vi "niFpgaMeanVarStdOutsideSCTL.vi"(0 "input data":fxp<+/-,32,1>, 1 "reset":bool) -> (4 "mean":fxp<+/-,32,1> format="%.32g", 6 "standard deviation":fxp<+,32,1> format="%.32g", 8 "variance":fxp<+,63,1> format="%.63g", 10 "output valid":bool)   [LabVIEW 2017]
doc: "Calculates the <B>DC (Mean)</B> and/or <B>RMS</B> values of an input signal. You also can use this VI to calculate the intermediate <B>Sum</B>, <B>Mean Square</B>, and <B>Square Sum</B> values in order to save FPGA resources."
uses:
  <vilib>/rvi/FXPMathLib/basic elements/FxpIntAccumulator/XNode/nifxpmath_IntAccumulator.xnode
  <vilib>/rvi/FXPMathLib/basic elements/FxpIntAccumulator/simVIs/DllFxpIntAccumulator_sub.vi
  <vilib>/rvi/FXPMathLib/basic elements/FxpIntAccumulator/subVIs/nifxpmath_IntAccumulator_SimConfig.ctl
  <vilib>/rvi/FXPMathLib/FxpMul/XNode/nifxpmath_Multiplier.xnode
  <vilib>/fxp/LVFixedPointOverflowPolicyTypeDef.ctl
  <vilib>/rvi/FXPMathLib/FxpSqrt/XNode/nifxpmath_Sqrt.xnode
  <vilib>/Platform/TimedLoop/XDataNode/XDataNode.xnode
  <vilib>/Platform/TimedLoop/XDataNode/nitl_modes.ctl
  <vilib>/Platform/TimedLoop/XDataNode/XDNodeRunTimeDep.lvlib
  <vilib>/Platform/TimedLoop/XDataNode/wakeup.ctl
  <vilib>/Platform/TimedLoop/XDataNode/timing_clust.ctl
  <vilib>/rvi/FXPMathLib/FxpSqrt/simVIs/DllSqrtTemp_sub.vi
  <vilib>/rvi/FXPMathLib/FxpSqrt/subVIs/nifxpmath_Sqrt_SimConfig.ctl
  <vilib>/rvi/FXPMathLib/sim/FxpSim.dll
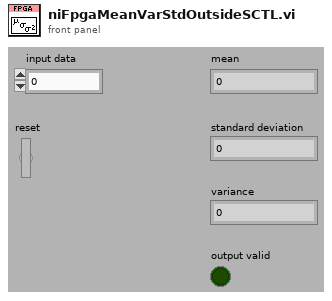
[diagram p1: front panel]
types:
  T1 = typedef "XDNodeRunTimeDep.lvlib/timing_clust.ctl" = cluster{"Expected End [f-1]":u64, "Actual End [f-1]":u64, "Finished Late? [f-1]":bool, "Expected End [i-1]":u64, "Actual End [i-1]":u64, "Finished Late? [i-1]":bool, "Expected Start [i]":u64, "Actual Start [i]":u64, "Expected Start [f]":u64, "Actual Start [f]":u64, "Source Name":string, "Structure Name":string, "Period":i64, "Deadline":i64, "Offset":i64, "Start":i64, "Priority":i32, "Timeout":i32, "Mode":T2, "Wakeup Reason":T3, "Error":errorcluster, "Source Type":string, "Secondary Source Type":string, "Global End Time":u64, "Global Start Time":u64, "Frame Duration":u64, "Iteration Duration":u64, "Assigned CPU":i32, "I/O Scan Engine Mode":u32}
  T2 = typedef "XDNodeRunTimeDep.lvlib/nitl_modes.ctl" = enum32{"No Change", "Process missed periods, maintain original phase", "Discard missed periods, maintain original phase", "Process missed periods, ignore original phase", "Discard missed periods, ignore original phase"}
  T3 = typedef "XDNodeRunTimeDep.lvlib/wakeup.ctl" = enum32{"Normal", "Aborted", "Asynchronous wakeup", "Timing source error", "Timed loop error", "Timeout"}
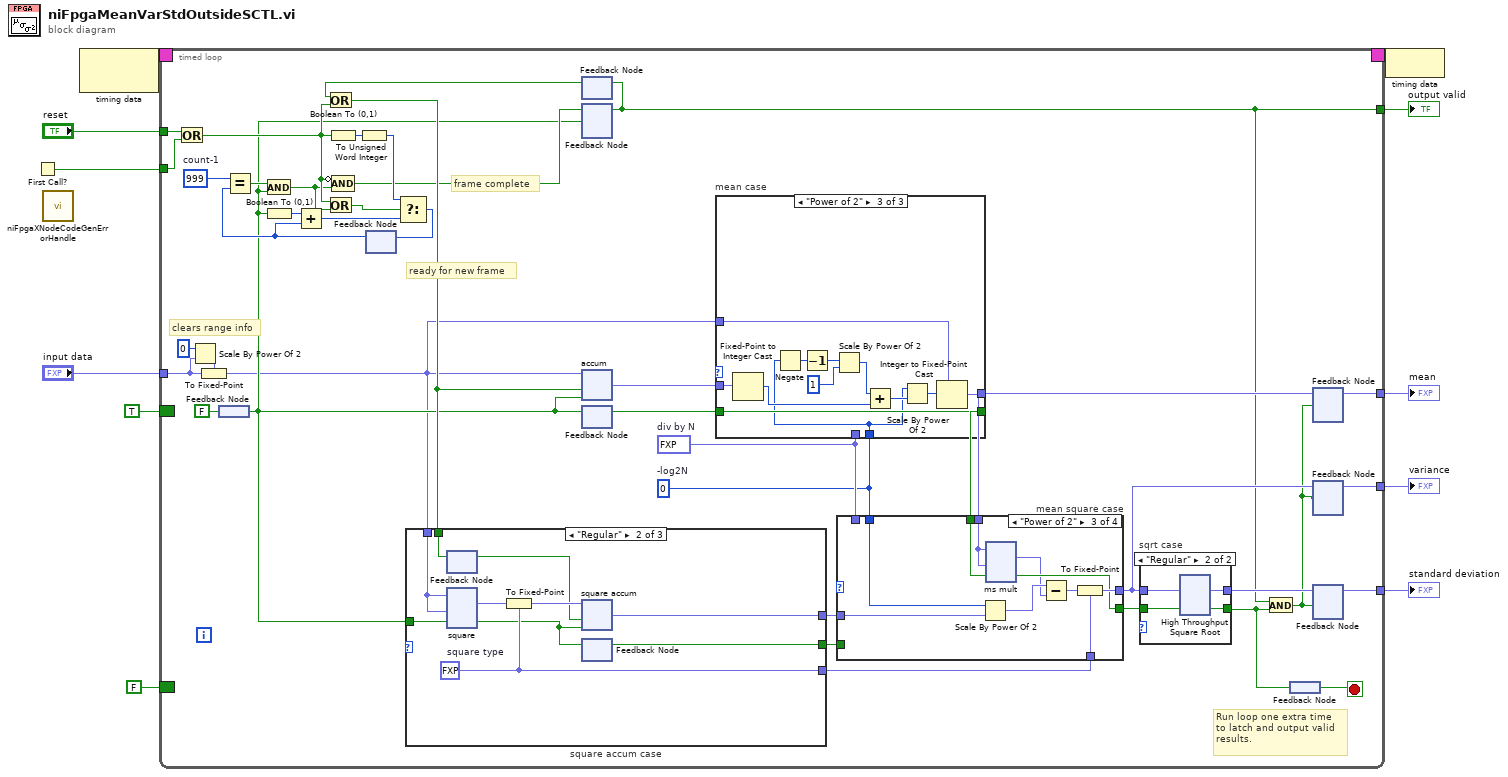
[diagram p0: block diagram]
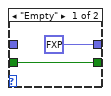
[diagram p2: hidden frame]
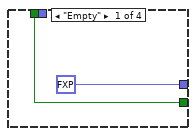
[diagram p3: hidden frame]
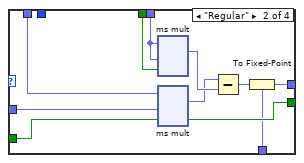
[diagram p4: hidden frame]
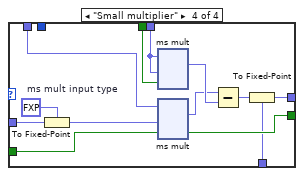
[diagram p5: hidden frame]
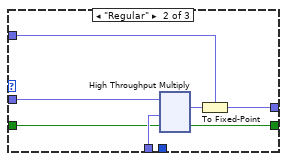
[diagram p7: hidden frame]
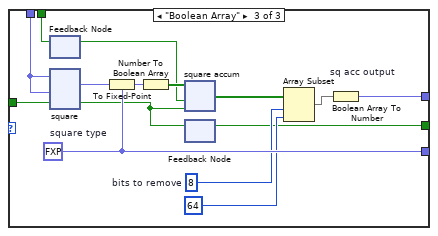
[diagram p9: hidden frame]
diagram:
  n1 = First Call?() -> (First Call?: T/F=w10:bool)
  n2 = call <vilib>:"niFpgaXNodeCodeGenErrorHandle.vi"() -> ()  [unwired: 1 in]
  n3 = node-c288() -> (w9:T1)  [unwired: 1 in]
  n4 = timed-loop {
    tunnel: [w22] -> w4
    tunnel: "input data" -> [w13]
    tunnel: "reset" -> [w48]
    tunnel: w10 -> [w47]
    tunnel: [w20] -> w3
    tunnel: [w18] -> w2
    tunnel: [w17] -> w7
    timing: w9 -> [_]
    timing-out: [_] -> w8
    border: TRUE -> [_]
    border: FALSE ("output valid") -> [_]
    stop <- w14 stop-if-true
    w31 = i8 0  # -log2N
    w37 = fxp<+,17,-9> 0.0010000020265579224  # div by N
    w52 = u16 999  # count-1
    # "Run loop one extra time\nto latch and output valid\nresults."
    # "clears range info"
    # "frame complete"
    # "ready for new frame"
    n5 = Or(x=w48, y=w47) -> (x .or. y?=w42:bool)
    n6 = Scale By Power Of 2(n=0, x=w13) -> (x*2^n=w26:fxp<+/-,32,1>)
    n7 = To Fixed-Point(fixed-point type=w26, number=w13) -> (fixed-point=w12:fxp<+/-,32,1>)
    n8 = feedback #1() -> (w24:bool)
    n9 = feedback-in #1(FALSE) -> ()
    n10 = Boolean To (0,1)(Boolean=w24) -> (0, 1=w46:i16)
    n11 = Boolean To (0,1)(Boolean=w42) -> (0, 1=w51:i16)
    n12 = To Unsigned Word Integer(number=w51) -> (unsigned 16bit integer=w50:u16)
    n13 = feedback #2() -> (w39:u16)  [unwired: 1 in]
    n14 = Equal?(x=w52, y=w39) -> (x = y?=w44:bool)
    n15 = And(x=w44, y=w24) -> (x .and. y?=w41:bool)
    n16 = Add(x=w46, y=w39) -> (x+y=w45:u16)
    n17 = Or(x=w42, y=w41) -> (x .or. y?=w43:bool)
    n18 = Compound Arithmetic op=AND(invert w42, w41) -> (w33:bool)
    n19 = Select(t=w50, s=w43, f=w45) -> (s? t:f=w49:u16)
    n20 = feedback-in #2(w49) -> ()
    n21 = feedback #3() -> (w40:bool)  [unwired: 1 in]
    n22 = Or(x=w40, y=w42) -> (x .or. y?=w35:bool)
    n23 = case "square accum case" shown="\"Regular\"" {
      selector: _ -> [_ _ _]
      tunnel: w12 -> [_ w173 w216]
      tunnel: w24 -> [_ w167 w206]
      tunnel: w35 -> [_ w169 w204]
      tunnel: [_ w172 w208] -> w32
      tunnel: [_ w171 w215] -> w34
      tunnel: [_ w170 w207] -> w29
      frame "Empty" {
      }
      frame "Regular" {
        w171 = fxp<+,63,1> 0.0  # square type
        n24 = feedback-in #4(w169) -> ()
        n25 = feedback #4() -> (w168:bool)  [unwired: 1 in]
        n26 = xnode ("square")("x"=w173, "y"=w173, "input valid"=w167) -> ("x*y"=w175:fxp<+/-,64,2>, "output valid"=w166:bool)  [unwired: 1 in, 1 out]
        n27 = To Fixed-Point(fixed-point type=w171, number=w175) -> (fixed-point=w174:fxp<+,63,1>)
        n28 = xnode "square accum"("x"=w174, "load (F)"=w168, "enable (T)"=w166) -> ("s"=w172:fxp<+,63,1>)  [unwired: 2 in, 1 out]
        n29 = feedback-in #5(w166) -> ()
        n30 = feedback #5() -> (w170:bool)  [unwired: 1 in]
      }
      frame "Boolean Array" {
        w212 = 8  # bits to remove
        w215 = fxp<+,63,1> 0.0  # square type
        n31 = feedback-in #6(w204) -> ()
        n32 = feedback #6() -> (w203:bool)  [unwired: 1 in]
        n33 = xnode ("square")("x"=w216, "y"=w216, "input valid"=w206) -> ("x*y"=w217:fxp<+/-,64,2>, "output valid"=w205:bool)  [unwired: 1 in, 1 out]
        n34 = To Fixed-Point(fixed-point type=w215, number=w217) -> (fixed-point=w214:fxp<+,63,1>)
        n35 = Number To Boolean Array(number=w214) -> (Boolean array=w213:bool[])
        n36 = xnode "square accum"("x"=w213, "load (F)"=w203, "enable (T)"=w205) -> ("s"=w209:bool[])  [unwired: 2 in, 1 out]
        n37 = feedback-in #7(w205) -> ()
        n38 = feedback #7() -> (w207:bool)  [unwired: 1 in]
        n39 = Array Subset(array=w209, index=w212, length=64) -> (w210:bool[])
        n40 = Boolean Array To Number "sq acc output"(Boolean array=w210) -> (number=w208:fxp<+,64,11>)
      }
    }
    n41 = feedback-in #8(w33, w24) -> ()
    n42 = feedback #8() -> (w17:bool)  [unwired: 1 in]
    n43 = feedback-in #3(w17) -> ()
    n44 = xnode "accum"("x"=w12, "load (F)"=w35, "enable (T)"=w24) -> ("s"=w36:fxp<+/-,42,11>)  [unwired: 2 in, 1 out]
    n45 = feedback-in #9(w24) -> ()
    n46 = feedback #9() -> (w30:bool)  [unwired: 1 in]
    n47 = case "mean case" shown="\"Power of 2\"" {
      selector: _ -> [_ _ _]
      tunnel: [_ w153 w155] -> w23
      tunnel: w37 -> [_ w151 _]
      tunnel: w36 -> [_ w150 w158]
      tunnel: w12 -> [_ w149 w157]
      tunnel: w30 -> [w146 w148 w165]
      tunnel: w31 -> [_ _ w154]
      tunnel: [w146 w147 w165] -> w28
      frame "Empty" {
      }
      frame "Regular" {
        n48 = xnode "High Throughput Multiply"("x"=w150, "y"=w151, "input valid"=w148) -> ("x*y"=w152:fxp<+/-,59,2>, "output valid"=w147:bool)  [unwired: 1 in, 1 out]
        n49 = To Fixed-Point(fixed-point type=w149, number=w152) -> (fixed-point=w153:fxp<+/-,32,1>)
      }
      frame "Power of 2" {
        n50 = Fixed-Point to Integer Cast(1:w158) -> (0:w160:i64)
        n51 = Negate(x=w154) -> (-x=w164:i8)
        n52 = Decrement(x=w164) -> (x-1=w163:i8)
        n53 = Scale By Power Of 2(n=w163, x=i64 1 ("x-1")) -> (x*2^n=w161:i64)
        n54 = Add(x=w161, y=w160) -> (x+y=w156:i64)
        n55 = Scale By Power Of 2(n=w154, x=w156) -> (x*2^n=w159:i64)
        n56 = Integer to Fixed-Point Cast(fixed-point type=w157, integer=w159) -> (fixed-point=w155:fxp<+/-,32,1>)
      }
    }
    n57 = case "mean square case" shown="\"Power of 2\"" {
      selector: _ -> [_ _ _ _]
      tunnel: [w111 w122 w125 w145] -> w38
      tunnel: w37 -> [_ w121 _ w144]
      tunnel: [fxp<+,63,1> 0.0 ("square type") w120 w132 w143] -> w21
      tunnel: w34 -> [_ w119 w131 w142]
      tunnel: w32 -> [_ w118 w129 w141]
      tunnel: w31 -> [_ _ w130 _]
      tunnel: w29 -> [_ w117 _ w138]
      tunnel: w23 -> [_ w116 w128 w137]
      tunnel: w28 -> [w111 w115 w127 w136]
      frame "Empty" {
      }
      frame "Regular" {
        n58 = xnode ("ms mult")("x"=w116, "y"=w116, "input valid"=w115) -> ("x*y"=w114:fxp<+/-,64,2>)  [unwired: 1 in, 2 out]
        n59 = xnode ("ms mult")("x"=w121, "y"=w118, "input valid"=w117) -> ("x*y"=w113:fxp<+,64,2>, "output valid"=w122:bool)  [unwired: 1 in, 1 out]
        n60 = Subtract(x=w113, y=w114) -> (x-y=w112:fxp<+/-,64,4>)
        n61 = To Fixed-Point(fixed-point type=w119, number=w112) -> (fixed-point=w120:fxp<+,63,1>)
      }
      frame "Power of 2" {
        n62 = Scale By Power Of 2(n=w130, x=w129) -> (x*2^n=w124:fxp<+,64,11>)
        n63 = xnode ("ms mult")("x"=w128, "y"=w128, "input valid"=w127) -> ("x*y"=w123:fxp<+/-,64,2>, "output valid"=w125:bool)  [unwired: 1 in, 1 out]
        n64 = Subtract(x=w124, y=w123) -> (x-y=w126:fxp<+/-,64,13>)
        n65 = To Fixed-Point(fixed-point type=w131, number=w126) -> (fixed-point=w132:fxp<+,63,1>)
      }
      frame "Small multiplier" {
        w139 = fxp<+,34,10> 0.0  # ms mult input type
        n66 = To Fixed-Point(fixed-point type=w139, number=w141) -> (fixed-point=w140:fxp<+,34,10>)
        n67 = xnode ("ms mult")("x"=w137, "y"=w137, "input valid"=w136) -> ("x*y"=w135:fxp<+/-,64,2>)  [unwired: 1 in, 2 out]
        n68 = xnode ("ms mult")("x"=w144, "y"=w140, "input valid"=w138) -> ("x*y"=w134:fxp<+,51,1>, "output valid"=w145:bool)  [unwired: 1 in, 1 out]
        n69 = Subtract(x=w134, y=w135) -> (x-y=w133:fxp<+/-,64,3>)
        n70 = To Fixed-Point(fixed-point type=w142, number=w133) -> (fixed-point=w143:fxp<+,63,1>)
      }
    }
    n71 = case "sqrt case" shown="\"Regular\"" {
      selector: _ -> [_ _]
      tunnel: [fxp<+,32,1> 0.0 ("square type") w85] -> w19
      tunnel: [w81 w84] -> w15
      tunnel: w38 -> [w81 w83]
      tunnel: w21 -> [_ w82]
      frame "Empty" {
      }
      frame "Regular" {
        n72 = xnode "High Throughput Square Root"("x"=w82, "input valid"=w83) -> ("sqrt(x)"=w85:fxp<+,32,1>, "output valid"=w84:bool)  [unwired: 1 in, 1 out]
      }
    }
    n73 = And(x=w17, y=w15) -> (x .and. y?=w16:bool)
    n74 = feedback-in #10(w15) -> ()
    n75 = feedback #10() -> (w14:bool)
    n76 = feedback #11() -> (w22:fxp<+/-,32,1>)  [unwired: 1 in]
    n77 = feedback-in #11(w23, w16) -> ()
    n78 = feedback #12() -> (w20:fxp<+,63,1>)  [unwired: 1 in]
    n79 = feedback-in #12(w21, w16) -> ()
    n80 = feedback #13() -> (w18:fxp<+,32,1>)  [unwired: 1 in]
    n81 = feedback-in #13(w19, w16) -> ()
  }
  "output valid" <- w7
  "mean" <- w4
  "variance" <- w3
  "standard deviation" <- w2
  n82 = node-c288(w8) -> ()
